vi "ReadSubpanels.vi"(8 "error in (no error)":errorcluster, 11 "EmbeddedMainUI in":refnum<class "EmbeddedMainUI.lvclass">) -> (0 "error out":errorcluster, 2 "Subpanels":refnum<class "EmbeddedSMO.lvclass">[](array[class]), 3 "EmbeddedMainUI out":refnum<class "EmbeddedMainUI.lvclass">)   [LabVIEW 2016, in "EmbeddedMainUI.lvclass"]
uses:
  EmbeddedMainUI.lvclass
  <vilib>/Levylab/Embedded SMO UI/EmbeddedSMO.lvclass
  EmbeddedMainUI.lvclass/EmbeddedMainUI.ctl
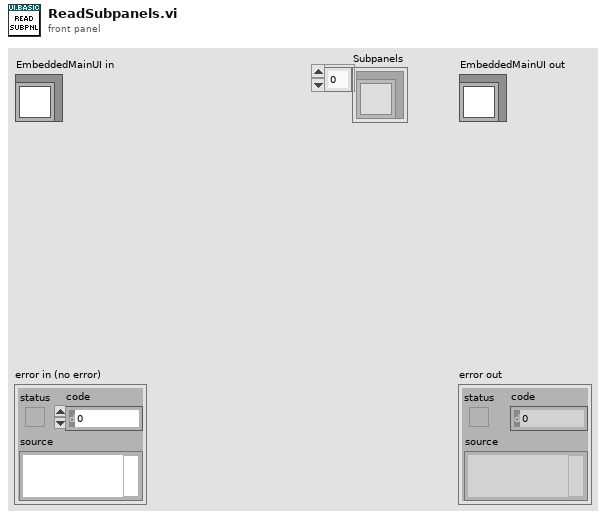
[diagram p1: front panel]
types:
  T1 = typedef "EmbeddedMainUI.lvclass/FrameworkDataRef.ctl" = refnum<data-value>
  T2 = typedef "EmbeddedMainUI.lvclass/FrameworkData.ctl" = cluster{"Subpanels":refnum<class "EmbeddedSMO.lvclass">[], "Left Subpanel":refnum<vi>, "Right Subpanel":refnum<vi>, "Active Left":i32, "Active Right":i32}
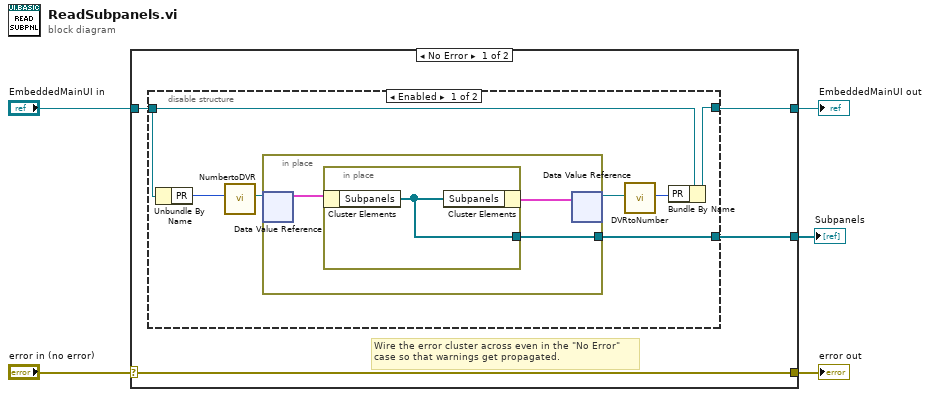
[diagram p0: block diagram]
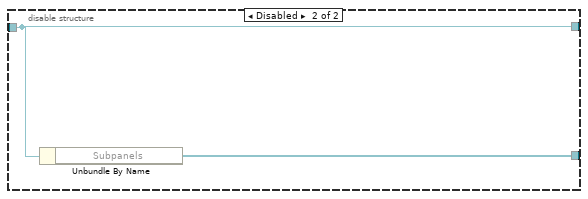
[diagram p2: hidden frame]
diagram:
  n1 = case shown="No Error" "error in (no error)" {
    selector: "error in (no error)" -> [w9 w24]
    tunnel: [w9 w24] -> w4
    tunnel: [w7 w23] -> w2
    tunnel: "EmbeddedMainUI in" -> [w8 w23]
    tunnel: [w6 _] -> w1
    frame No Error {
      # "Wire the error cluster across even in the \"No Error\"\ncase so that warnings get propagated."
      n2 = disable-structure shown="Enabled" {
        disable-tunnel: w8 -> [w16 w21]
        disable-tunnel: [w14 w21] -> w7
        disable-tunnel: [w15 w22] -> w6
        frame Enabled {
          n3 = Unbundle By Name(w16) -> ("PR"=w13:i32)
          n4 = call "NumbertoDVR.vi"("Numeric"=w13) -> ("FrameworkDataRef"=w12:T1)  [unwired: 10 in]
          n5 = in-place {
            in-place-border: [w17] -> w15
            n6 = in-place-dvr #1(w12) -> (w19:T2)  [unwired: 1 out]
            n7 = in-place {
              in-place-border: [w20] -> w17
              n8 = in-place-cluster #2(w19) -> ("Subpanels"=w20:refnum<class "EmbeddedSMO.lvclass">[])
              n9 = in-place-cluster #2("Subpanels"=w20) -> (w18:T2)
            }
            n10 = in-place-dvr #1(w18) -> (w11:T1)  [unwired: 1 out]
          }
          n11 = call "DVRtoNumber.vi"("FrameworkDataRef"=w11) -> ("Number"=w10:i32)  [unwired: 10 in]
          n12 = Bundle By Name(cluster=w16, "PR"=w10) -> (w14:refnum<class "EmbeddedMainUI.lvclass">)
        }
        frame Disabled {
          n13 = Unbundle By Name(w21) -> ("Subpanels"=w22:refnum<class "EmbeddedSMO.lvclass">[])
        }
      }
    }
    frame Error {
    }
  }
  "error out" <- w4
  "EmbeddedMainUI out" <- w2
  "Subpanels" <- w1
